vi "Ease Menu Buttons.vi"(8 "error in (no error)":errorcluster, 11 "User Interface References":T1) -> (0 "error out":errorcluster)   [LabVIEW 2011, in "Sliding Menu Library.lvlib"]
uses:
  Sliding Menu Library.lvlib
  <vilib>/Utility/config.llb/Config Data RefNum.ctl
  <vilib>/Utility/config.llb/NI_LVConfig.lvlib
  Sliding Menu Type Definitions/User Interface Type Definitions.ctl
  Button XControl.xctl
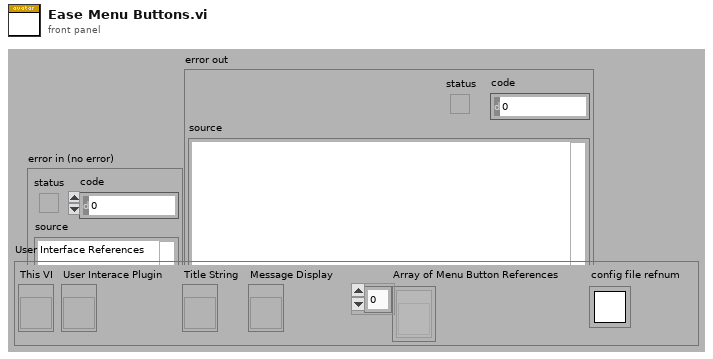
[diagram p1: front panel]
types:
  T1 = typedef "Sliding Menu Library.lvlib/User Interface Type Definitions.ctl" = cluster{"This VI":refnum<vi>, "User Interace Plugin":refnum<vi>, "Title String":refnum<vi>, "Message Display":refnum<vi>, "Array of Menu Button References":refnum<vi>[], "config file refnum":T2}
  T2 = typedef "NI_LVConfig.lvlib/Config Data RefNum.ctl" = refnum<k1>
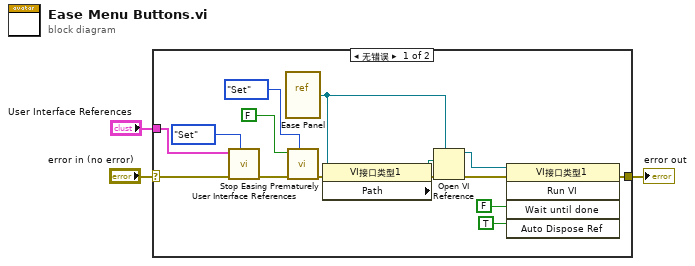
[diagram p0: block diagram]
diagram:
  n1 = case shown="无错误" "error in (no error)" {
    selector: "error in (no error)" -> [w12 w19]
    tunnel: [w13 w19] -> w3
    tunnel: "User Interface References" -> [w11 _]
    frame No Error {
      n2 = call "User Interface References.vi"("Set or Get Value"=enum16{"Set", "Get"}."Set", "error in"=w12, "User Interface References"=w11) -> ("error out"=w7:errorcluster)  [unwired: 7 in, 1 out]
      n3 = vi-ref "Ease Panel.vi"() -> (w5:refnum<vi>)
      n4 = call "Stop Easing Prematurely.vi"("Set or Get Value"=enum16{"Set", "Get"}."Set", "error in"=w7, "Stop?"=FALSE) -> ("error out"=w6:errorcluster)  [unwired: 7 in, 1 out]
      n5 = property class="VI接口类型1"(reference=w5, error in=w6) -> (error out=w15:errorcluster, "Path"=w18:path)  [unwired: 1 out]
      n6 = Open VI Reference(type specifier VI Refnum (for type only)=w5, vi path=w18, error in (no error)=w15) -> (vi reference=w17:refnum<vi>, error out=w14:errorcluster)  [unwired: 3 in]
      n7 = invoke class="VI接口类型1" method="Run VI"(reference=w17, error in=w14, "Wait until done"=FALSE ("Wait Until Done"), "Auto Dispose Ref"=TRUE ("Auto Dispose Reference")) -> (error out=w13:errorcluster)  [unwired: 1 in, 4 out]
    }
    frame Error {
    }
  }
  "error out" <- w3
